vi "pressure Realease.vi"(7 "init":bool, 8 "error in (no error)":errorcluster, 10 "Direction":T1, 11 "Stand in":refnum<class "Stand.lvclass">) -> (0 "error out":errorcluster, 2 "done":bool, 3 "Stand out":refnum<class "Stand.lvclass">)   [LabVIEW 2019, in "Stand.lvclass"]
uses:
  Stand.lvclass
  TypeDef/Direction.ctl
  D:/GIT H4000/H4000/src/Device_class/Device.lvclass
  Stand.lvclass/Stand.ctl
  Device_class/Device.lvclass/Device.ctl
  AI_class/AI.lvclass/AI.ctl
  AnalogComparator_class/AnalogComparator.lvclass/AnalogComparator.ctl
  dY_dX_Calculator/delayValue.lvclass/delayValue.ctl
  FPGA/TypeDef/DO index.ctl
  NeedleValve_class/Cmd.ctl
  AnalogComparator_class/GetStatus.vi
  FPGA_API_class/FPGA API.lvclass
  Device_class/Device.lvclass
  AI_class/AI.lvclass
  dY_dX_Calculator/delayValue.lvclass
  NeedleValve_class/NeedleValve.lvclass
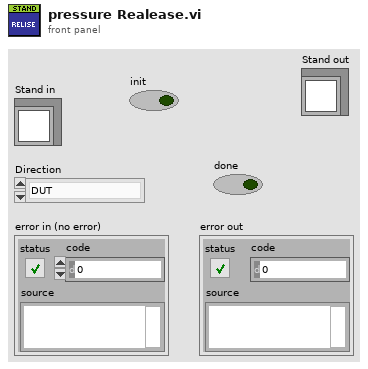
[diagram p1: front panel]
types:
  T1 = typedef "Direction.ctl" = enum8{"DUT", "Chamber"}
  T2 = typedef "NeedleValve.lvclass/Cmd.ctl" = enum16{"Open", "Close", "Stop", "Prep open"}
  T3 = typedef "AI_Data.ctl" = cluster{"Stat Data":T4, "OutOfRangeMax":bool, "OutOfRangeMin":bool, "HIHI":bool, "HI":bool, "LO":bool, "LOLO":bool}
  T4 = typedef "AI Statistics Data.ctl" = cluster{"raw mean":dbl, "scl mean":dbl, "raw mean 1Hz":dbl, "scl mean 1Hz":dbl}
  T5 = typedef "Setting Pressure PI.ctl" = cluster{"A [MPa/V]":dbl, "P0 [MPa]":dbl}
  T6 = typedef "DO index.ctl" = u8
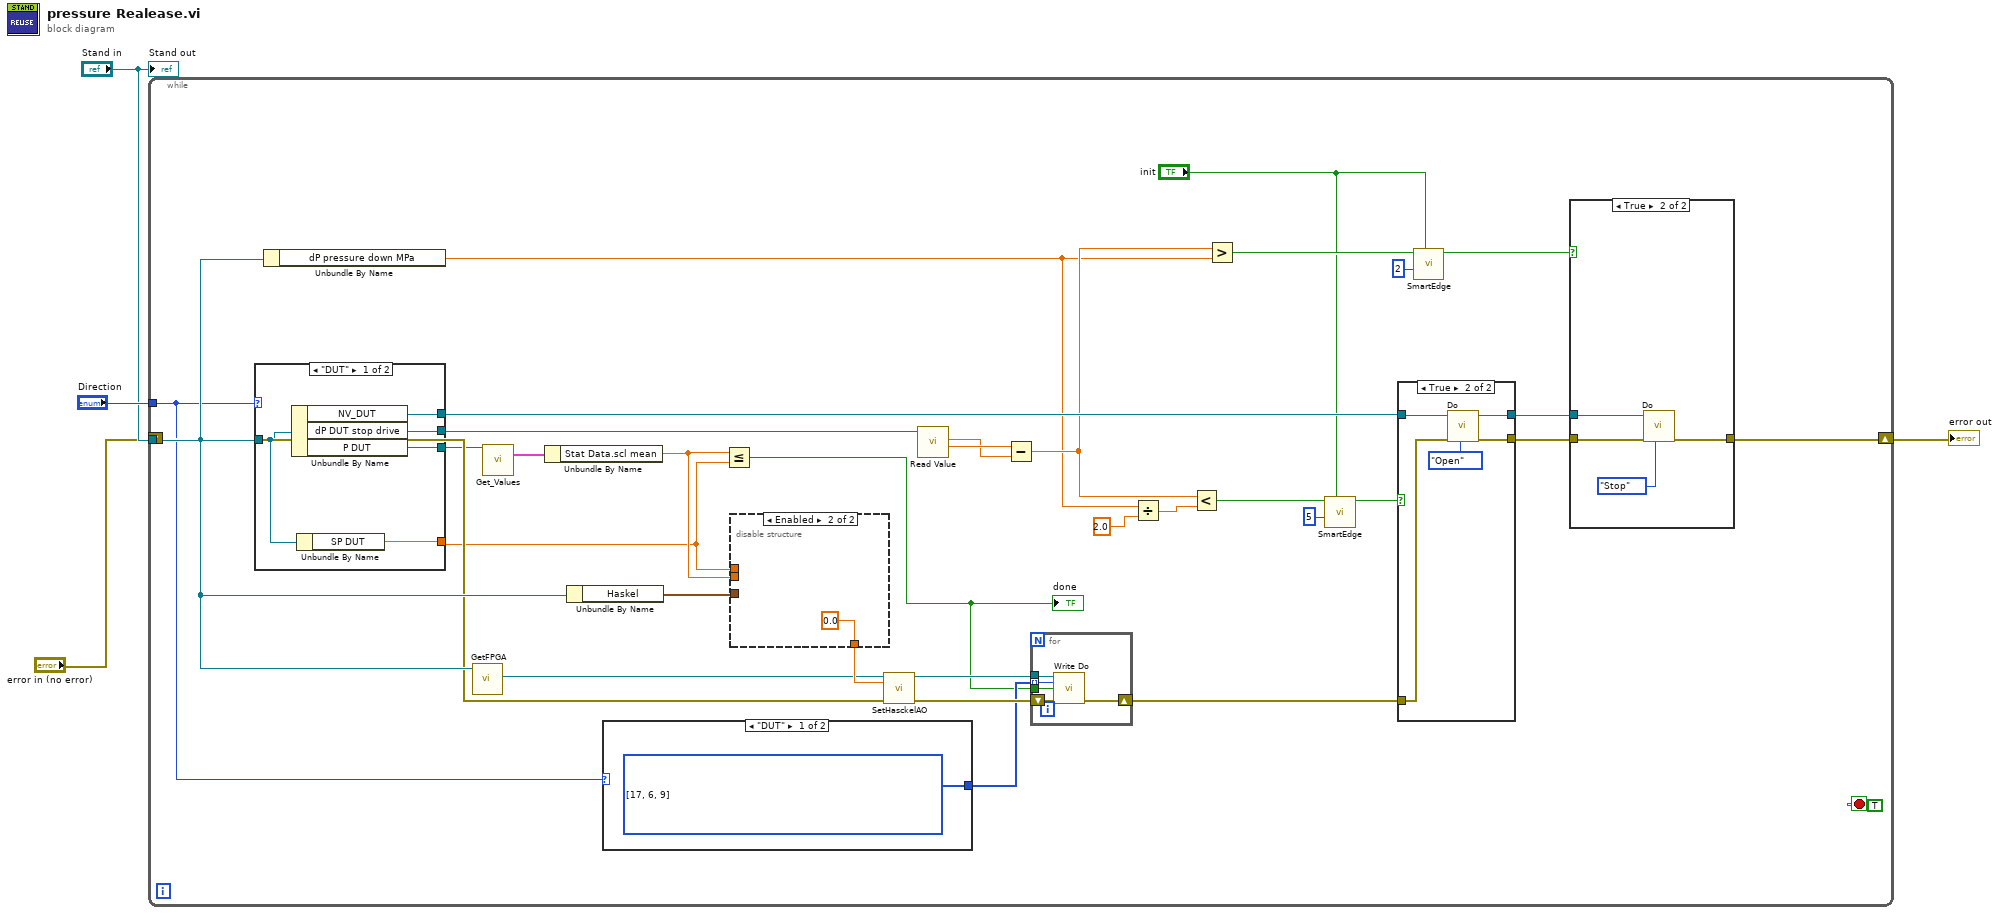
[diagram p0: block diagram]
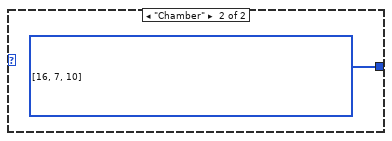
[diagram p2: hidden frame]
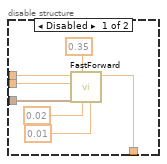
[diagram p3: hidden frame]
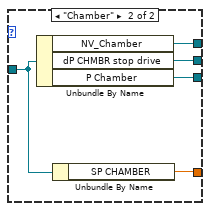
[diagram p4: hidden frame]
diagram:
  n1 = while {
    tunnel: "Direction" -> [w8]
    tunnel: "Stand in" -> [w38]
    shift-right: [w14] -> w2
    shift-left: "error in (no error)" -> [w37]
    stop <- TRUE stop-if-true
    n2 = case shown="\"DUT\"" w8 {
      tunnel: w38 -> [w55 w60]
      tunnel: [w58 w63] -> w32
      tunnel: [w57 w62] -> w30
      tunnel: [w56 w61] -> w26
      tunnel: [w54 w59] -> w25
      frame "DUT" {
        n3 = Unbundle By Name(w55) -> ("NV_DUT"=w56:refnum<class "NeedleValve.lvclass">, "dP DUT stop drive"=w57:refnum<class "delayValue.lvclass">, "P DUT"=w58:refnum<class "AI.lvclass">)
        n4 = Unbundle By Name(w55) -> ("SP DUT"=w54:dbl)
      }
      frame "Chamber" {
        n5 = Unbundle By Name(w60) -> ("NV_Chamber"=w61:refnum<class "NeedleValve.lvclass">, "dP CHMBR stop drive"=w62:refnum<class "delayValue.lvclass">, "P Chamber"=w63:refnum<class "AI.lvclass">)
        n6 = Unbundle By Name(w60) -> ("SP CHAMBER"=w59:dbl)
      }
    }
    n7 = Unbundle By Name(w38) -> ("dP pressure down MPa"=w21:dbl)
    n8 = call "GetFPGA.vi"("Device in"=w38) -> ("FPGA API.lvclass"=w31:refnum<class "FPGA API.lvclass">)  [unwired: 10 in]
    n9 = call "Get_Values.vi"("reference in"=w32) -> ("Data"=w35:T3)  [unwired: 14 in]
    n10 = Unbundle By Name(w35) -> ("Stat Data.scl mean"=w33:dbl)
    n11 = Unbundle By Name(w38) -> ("Haskel"=w27:T5)
    n12 = case shown="\"DUT\"" w8 {
      tunnel: [w39 w40] -> w9
      frame "DUT" {
        w39 = T6[] [17, 6, 9] items=["DO 0 [KP1] [M12]", "DO 1 [ON KP2] [M21]", "DO 2 [ON KP3] [M24]", "DO 3 [WATER Y18.1 [DO3]]", "DO 4 [WATER Y18.2 [DO4]]", "DO 5 [KP6 Y29.1 33.7]", "DO 6 [KP7 Y29.2 33.8]", "DO 7 [KP8 Y29.3 33.9]", "DO 8 [KP9 Y29.4  33.12]", "DO 9 [KP10 Y29.5 33.1]", "DO 10 [KP11 Y29.6 33.2]", "DO 11 [KP12 Y29.7  33.13]", "DO 12 [KP13 Y29.8  33.11]", "DO 13 [KP14 Y29.9 33.10]", "DO 14 [KP15 Y29.10  33.6]", "DO 15 [KP16 Y29.11  33.5]", "DO 16 [KP17 Y29.12  33.4]", "DO 17 [KP18 Y29.13 33.3]", "DO 18 [AIR KP19]", "DO 19 [STEP DRIVE EN KP20]", "DO 20 [KP21 Y44.1 OPEN]", "DO 21 [ KP22 Y44.1 CLOSE]", "DO 22 [ KP23 Y44.2 OPEN]", "DO 23", "DO 24 [STEP DRIVE 1]", "DO 25 [STEP DRIVE 2]"] ("#DO")
      }
      frame "Chamber" {
        w40 = T6[] [16, 7, 10] items=["DO 0 [KP1] [M12]", "DO 1 [ON KP2] [M21]", "DO 2 [ON KP3] [M24]", "DO 3 [WATER Y18.1 [DO3]]", "DO 4 [WATER Y18.2 [DO4]]", "DO 5 [KP6 Y29.1 33.7]", "DO 6 [KP7 Y29.2 33.8]", "DO 7 [KP8 Y29.3 33.9]", "DO 8 [KP9 Y29.4  33.12]", "DO 9 [KP10 Y29.5 33.1]", "DO 10 [KP11 Y29.6 33.2]", "DO 11 [KP12 Y29.7  33.13]", "DO 12 [KP13 Y29.8  33.11]", "DO 13 [KP14 Y29.9 33.10]", "DO 14 [KP15 Y29.10  33.6]", "DO 15 [KP16 Y29.11  33.5]", "DO 16 [KP17 Y29.12  33.4]", "DO 17 [KP18 Y29.13 33.3]", "DO 18 [AIR KP19]", "DO 19 [STEP DRIVE EN KP20]", "DO 20 [KP21 Y44.1 OPEN]", "DO 21 [ KP22 Y44.1 CLOSE]", "DO 22 [ KP23 Y44.2 OPEN]", "DO 23", "DO 24 [STEP DRIVE 1]", "DO 25 [STEP DRIVE 2]"] ("#DO")
      }
    }
    n13 = Less Or Equal?(x=w33, y=w25) -> (x <= y?=w7:bool)
    "done" <- w7
    n14 = disable-structure shown="Enabled" {
      disable-tunnel: [w52 0.0 ("Haskel in")] -> w34
      disable-tunnel: w33 -> [w51 _]
      disable-tunnel: w27 -> [w50 _]
      disable-tunnel: w25 -> [w49 _]
      frame Disabled {
        n15 = call "FastForward.vi"("delta U [V]"=0.01, "Epsilon A"=0.02, "U min [V]"=0.35, "Setting"=w50, "PV"=w51, "SP"=w49) -> ("U"=w52:dbl)  [unwired: 5 in]
      }
      frame Enabled {
      }
    }
    n16 = call-dynamic "SetHasckelAO.vi"("FPGA API in"=w31, "Haskel in"=w34, "error in (no error)"=w37) -> ("FPGA API out"=w11:refnum<class "FPGA API.lvclass">, "error out"=w12:errorcluster)  [unwired: 11 in]
    n17 = call "Read Value.vi"("dY_dX_Calculator in"=w30) -> ("oldValue"=w29:dbl, "currValue"=w28:dbl)  [unwired: 9 in]
    n18 = Subtract(x=w29, y=w28) -> (x-y=w22:dbl)
    n19 = for {
      tunnel: w11 -> [w44]
      tunnel: w9 -> [w42] mode=indexing
      shift-right: [w43] -> w10
      shift-left: w12 -> [w45]
      tunnel: w7 -> [w41]
      n20 = call-dynamic "Write Do.vi"("FPGA API in"=w44, "#DO"=w42, "value"=w41, "error in (no error)"=w45) -> ("error out"=w43:errorcluster)  [unwired: 10 in, 1 out]
    }
    n21 = Divide(x=w21, y=2.0) -> (x/y=w23:dbl)
    n22 = Less?(x=w22, y=w23) -> (x < y?=w20:bool)
    n23 = Greater?(x=w22, y=w21) -> (0:w17:bool)
    n24 = call "SmartEdge.vi"("init"="init", "Filter Length"=5, "in"=w20) -> ("edge"=w19:bool)  [unwired: 8 in]
    n25 = case shown="True" w19 {
      tunnel: w26 -> [w69 w75]
      tunnel: w10 -> [w70 w74]
      tunnel: [w70 w73] -> w18
      tunnel: [w69 w71] -> w13
      frame False {
      }
      frame True {
        n26 = call "Do.vi"("Cmd"=Cmd."Open", "error in (no error)"=w74, "NeedleValve in"=w75) -> ("error out"=w73:errorcluster, "NeedleValve out"=w71:refnum<class "NeedleValve.lvclass">)  [unwired: 7 in]
      }
    }
    n27 = call "SmartEdge.vi"("init"="init", "Filter Length"=2, "in"=w17) -> ("edge"=w15:bool)  [unwired: 8 in]
    n28 = case shown="True" w15 {
      tunnel: [w64 w67] -> w14
      tunnel: w18 -> [w64 w66]
      tunnel: w13 -> [_ w65]
      frame False {
      }
      frame True {
        n29 = call "Do.vi"("Cmd"=Cmd."Stop", "error in (no error)"=w66, "NeedleValve in"=w65) -> ("error out"=w67:errorcluster)  [unwired: 7 in, 1 out]
      }
    }
  }
  "error out" <- w2
  "Stand out" <- "Stand in"
